vi "获取脚本.vi"(0 "Display State In":T2={"功能选择"=enum."扫描", "数据库引用"=refnum, "扫描参数"={"+ V"=0.0, "+ Δ V"=0.0, "+ limit I"=0.01, "- V"=0.0, "- Δ V"=0.0, "- limit I"=0.01, "NPLC"=0.001, "模型"=FALSE}, "保持时间"={"V"=0.0, "limit I"=0.01, "T"=0.0, "ΔT"=0.0, "NPLC"=0.001}, "脉冲1"={"t0"=timestamp(0 s since 1904-01-01), "dt"=1.0, "Y"=[]}, "脉冲2"={"t0"=timestamp(0 s since 1904-01-01), "dt"=1.0, "Y"=[]}, "高速脉冲1"={"t0"=timestamp(0 s since 1904-01-01), "dt"=1.0, "Y"=[]}, "高速脉冲2"={"t0"=timestamp(0 s since 1904-01-01), "dt"=1.0, "Y"=[]}, "任意波形"={"t0"=timestamp(0 s since 1904-01-01), "dt"=1.0, "Y"=[]}} caption="显示状态输入" {"保持时间"."ΔT" min=0.5 max=100.0 step=0.1 format="%#_6ps"; "保持时间"."T" min=10.0 max=4294000.0 step=1.0 format="%#_6ps"; "保持时间"."NPLC" min=1.0 max=20.0 step=1.0; "保持时间"."limit I" min=1e-08 max=3.0 format="%#_6pA"; "保持时间"."V" min=-40.0 max=40.0 format="%#_6pV"; "扫描参数"."NPLC" min=0.001 max=25.0 step=0.001; "扫描参数"."- Δ V" min=5e-05 max=1.0 step=5e-05 format="%#_6pV"; "扫描参数"."+ Δ V" min=5e-05 max=1.0 step=5e-05 format="%#_6pV"; "扫描参数"."- V" min=-40.0 max=40.0 format="%#_6pV"; "扫描参数"."- limit I" min=1e-08 max=3.0 format="%#_6pA"; "扫描参数"."+ limit I" min=1e-08 max=3.0 format="%#_6pA"; "扫描参数"."+ V" min=-40.0 max=40.0 format="%#_6pV"}, 5 "方向":T1, 9 "Container State":T7 caption="容器状态", 11 "error in (no error)":errorcluster caption="错误输入（无错误）") -> (4 "Display State Out":T2={"功能选择"=enum."扫描", "数据库引用"=refnum, "扫描参数"={"+ V"=0.0, "+ Δ V"=0.0, "+ limit I"=0.01, "- V"=0.0, "- Δ V"=0.0, "- limit I"=0.01, "NPLC"=0.001, "模型"=FALSE}, "保持时间"={"V"=0.0, "limit I"=0.01, "T"=0.0, "ΔT"=0.0, "NPLC"=0.001}, "脉冲1"={"t0"=timestamp(0 s since 1904-01-01), "dt"=1.0, "Y"=[]}, "脉冲2"={"t0"=timestamp(0 s since 1904-01-01), "dt"=1.0, "Y"=[]}, "高速脉冲1"={"t0"=timestamp(0 s since 1904-01-01), "dt"=1.0, "Y"=[]}, "高速脉冲2"={"t0"=timestamp(0 s since 1904-01-01), "dt"=1.0, "Y"=[]}, "任意波形"={"t0"=timestamp(0 s since 1904-01-01), "dt"=1.0, "Y"=[]}} caption="显示状态输出" {"保持时间"."ΔT" min=0.5 max=100.0 step=0.1 format="%#_6ps"; "保持时间"."T" min=10.0 max=4294000.0 step=1.0 format="%#_6ps"; "保持时间"."NPLC" min=1.0 max=20.0 step=1.0; "保持时间"."limit I" min=1e-08 max=3.0 format="%#_6pA"; "保持时间"."V" min=-40.0 max=40.0 format="%#_6pV"; "扫描参数"."NPLC" min=0.001 max=25.0 step=0.001; "扫描参数"."- Δ V" min=5e-05 max=1.0 step=5e-05 format="%#_6pV"; "扫描参数"."+ Δ V" min=5e-05 max=1.0 step=5e-05 format="%#_6pV"; "扫描参数"."- V" min=-40.0 max=40.0 format="%#_6pV"; "扫描参数"."- limit I" min=1e-08 max=3.0 format="%#_6pA"; "扫描参数"."+ limit I" min=1e-08 max=3.0 format="%#_6pA"; "扫描参数"."+ V" min=-40.0 max=40.0 format="%#_6pV"}, 6 "Script":string, 15 "error out":errorcluster caption="错误输出")   [LabVIEW 2020, in "功能选择.xctl"]
uses:
  <vilib>/_xctls/Container State.ctl
  <vilib>/addons/database/Connection.llb/Conn ObjectReference.ctl
  <vilib>/_xctls/XControlSupport.lvlib
  <vilib>/addons/database/NI_Database_API.lvlib
panel:
  # "功能选择.xctl:方向属性.ctl添加构成方法参数的输入控件及显示控件。连接至连线板。不要删除已连接至连线板的输入控件及显示控件。\n\n如需设置该方法的参数，右键单击项目树中的对应项并选择“配置方法...”。"
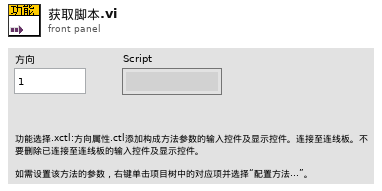
[diagram p1: front panel]
types:
  T1 = typedef "功能选择.xctl/方向属性.ctl" = enum16{"1", "2"}
  T2 = typedef "功能选择.xctl/状态.ctl" = cluster{"功能选择":T3, "数据库引用":T4, "扫描参数":T5, "保持时间":T6, "脉冲1":waveform(dbl), "脉冲2":waveform(dbl), "高速脉冲1":waveform(dbl), "高速脉冲2":waveform(dbl), "任意波形":waveform(dbl)}
  T3 = typedef "功能选择.xctl/功能类型选择.ctl" = enum16{"扫描", "循环扫描", "保持时间", "脉冲", "高速脉冲", "任意波形"}
  T4 = typedef "NI_Database_API.lvlib/Conn ObjectReference.ctl" = refnum<k1>
  T5 = typedef "功能选择.xctl/扫描参数.ctl" = cluster{"+ V":dbl, "+ Δ V":dbl, "+ limit I":dbl, "- V":dbl, "- Δ V":dbl, "- limit I":dbl, "NPLC":dbl, "模型":bool}
  T6 = typedef "功能选择.xctl/保持时间.ctl" = cluster{"V":dbl, "limit I":dbl, "T":dbl, "ΔT":dbl, "NPLC":dbl}
  T7 = typedef "XControlSupport.lvlib/Container State.ctl" = cluster{"Indicator?":bool, "Run Mode?":bool, " Refnum":refnum<vi>}
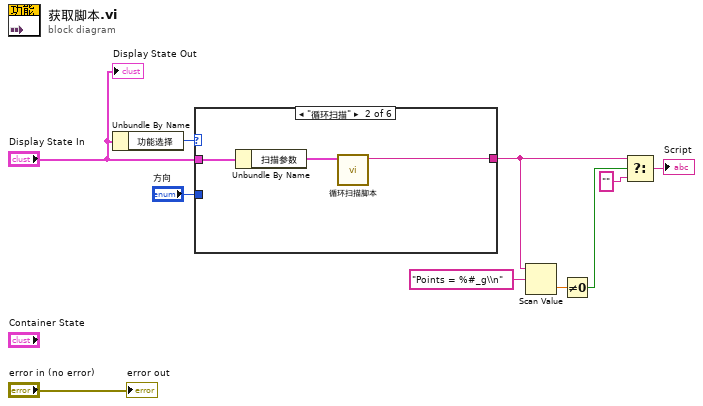
[diagram p0: block diagram]
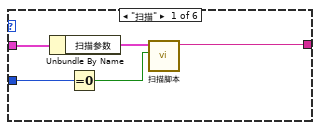
[diagram p2: hidden frame]
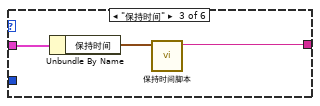
[diagram p3: hidden frame]
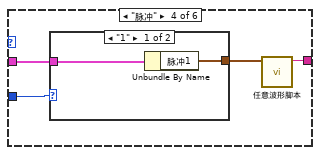
[diagram p4: hidden frame]
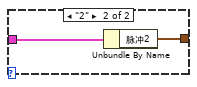
[diagram p5: hidden frame]
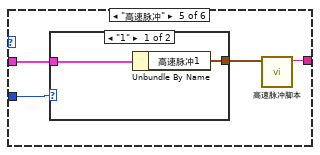
[diagram p6: hidden frame]
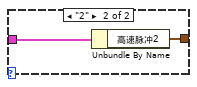
[diagram p7: hidden frame]
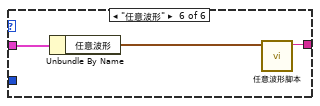
[diagram p8: hidden frame]
diagram:
  n1 = Unbundle By Name("Display State In") -> ("功能选择"=w9:T3)
  n2 = case shown="\"循环扫描\"" w9 {
    tunnel: "Display State In" -> [w15 w18 w21 w25 w33 w40]
    tunnel: [w14 w16 w19 w22 w30 w38] -> w2
    tunnel: "方向" -> [w12 _ _ w24 w32 _]
    frame "扫描" {
      n3 = Unbundle By Name(w15) -> ("扫描参数"=w13:T5)
      n4 = Equal To 0?(x=w12) -> (x = 0?=w11:bool)
      n5 = call "扫描脚本.vi"("方向(T:正向)"=w11, "扫描参数"=w13) -> ("Script"=w14:string)  [unwired: 9 in]
    }
    frame "循环扫描" {
      n6 = Unbundle By Name(w18) -> ("扫描参数"=w17:T5)
      n7 = call "循环扫描脚本.vi"("扫描参数"=w17) -> ("Script"=w16:string)  [unwired: 10 in]
    }
    frame "保持时间" {
      n8 = Unbundle By Name(w21) -> ("保持时间"=w20:T6)
      n9 = call "保持时间脚本.vi"("保持时间"=w20) -> ("Script"=w19:string)  [unwired: 10 in]
    }
    frame "脉冲" {
      n10 = case shown="\"1\"" w24 {
        tunnel: w25 -> [w27 w29]
        tunnel: [w26 w28] -> w23
        frame "1" {
          n11 = Unbundle By Name(w27) -> ("脉冲1"=w26:waveform(dbl))
        }
        frame "2" {
          n12 = Unbundle By Name(w29) -> ("脉冲2"=w28:waveform(dbl))
        }
      }
      n13 = call "任意波形脚本.vi"("波形"=w23) -> ("Script"=w22:string)  [unwired: 10 in]
    }
    frame "高速脉冲" {
      n14 = case shown="\"1\"" w32 {
        tunnel: w33 -> [w35 w37]
        tunnel: [w34 w36] -> w31
        frame "1" {
          n15 = Unbundle By Name(w35) -> ("高速脉冲1"=w34:waveform(dbl))
        }
        frame "2" {
          n16 = Unbundle By Name(w37) -> ("高速脉冲2"=w36:waveform(dbl))
        }
      }
      n17 = call "高速脉冲脚本.vi"("波形"=w31) -> ("Script"=w30:string)  [unwired: 10 in]
    }
    frame "任意波形" {
      n18 = Unbundle By Name(w40) -> ("任意波形"=w39:waveform(dbl))
      n19 = call "任意波形脚本.vi"("波形"=w39) -> ("Script"=w38:string)  [unwired: 10 in]
    }
  }
  n20 = Scan Value(string=w2, format string="Points = %#_g\\n" ("格式字符串")) -> (value=w5:dbl)  [unwired: 1 in, 1 out]
  n21 = Not Equal To 0?(x=w5) -> (x != 0?=w4:bool)
  n22 = Select(t=w2, s=w4, f="") -> (s? t:f=→"Script":string)
  "Display State Out" <- "Display State In"
  "error out" <- "error in (no error)"
